vi "Set Run ID.vi"(8 "error in (no error)":errorcluster, 11 "Sift Client in":refnum<class "Sift Client.lvclass">) -> (0 "error out":errorcluster, 3 "Sift Client out":refnum<class "Sift Client.lvclass">)   [LabVIEW 2024, in "Sift Client.lvlib" / "Sift Client.lvclass"]
doc: "Send the \"set_run_id\" Control message to Sift Proxy."
uses:
  Sift Client.lvclass
  Sift Client.lvclass/Sift Client.ctl
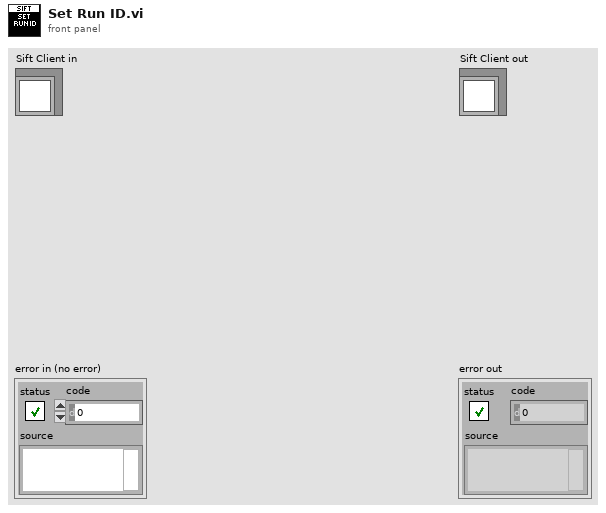
[diagram p1: front panel]
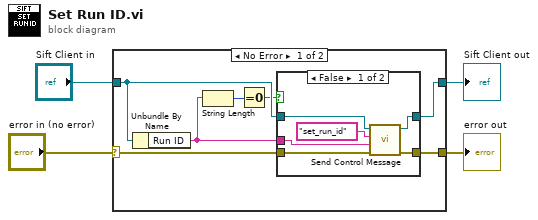
[diagram p0: block diagram]
diagram:
  n1 = case shown="No Error" "error in (no error)" {
    selector: "error in (no error)" -> [w11 w21]
    tunnel: [w9 w21] -> w3
    tunnel: [w8 w20] -> w1
    tunnel: "Sift Client in" -> [w10 w20]
    frame No Error {
      n2 = Unbundle By Name(w10) -> ("Run ID"=w5:string)
      n3 = String Length(string=w5) -> (length=w7:i32)
      n4 = Equal To 0?(x=w7) -> (x = 0?=w6:bool)
      n5 = case shown="False" w6 {
        tunnel: w5 -> [w12 _]
        tunnel: w11 -> [w17 w19]
        tunnel: w10 -> [w16 w18]
        tunnel: [w15 w19] -> w9
        tunnel: [w14 w18] -> w8
        frame False {
          n6 = call-dynamic "Send Control Message.vi"("error in (no error)"=w17, "Argument"=w12, "Command"="set_run_id", "Sift Client in"=w16) -> ("error out"=w15:errorcluster, "Sift Client out"=w14:refnum<class "Sift Client.lvclass">)  [unwired: 6 in]
        }
        frame True {
        }
      }
    }
    frame Error {
    }
  }
  "error out" <- w3
  "Sift Client out" <- w1
